vi "WILT.vi"() -> ()   [LabVIEW 2016] (continued)
"Temperature  Deg F (TC)"=0.0, "Volts"=0.0, "Volts (208)"=0.0, "SW (208)"=0.0}}, {"Lab ID"="", "Day Cycle Count"=0, "Station Label"="", "Dryer Details"={"Station"="", "Lab ID"="", "TR Number"=""}, "Status Color"=0, "Invisible Button"=FALSE, "Night Cycle Count"=0, "Station Index"=0, "Cycle Index"="", "Audit Alert"=FALSE, "Agilent Channel Definition"={"Channel"="", "Station"="", "Label"="", "Agilent Station"="", "Data"=0.0}, "DAQ Data"={"L1 Current"=0.0, "L2 Current"=0.0, "Temperature  Deg F (TC)"=0.0, "Volts"=0.0, "Volts (208)"=0.0, "SW (208)"=0.0}}, {"Lab ID"="", "Day Cycle Count"=0, "Station Label"="", "Dryer Details"={"Station"="", "Lab ID"="", "TR Number"=""}, "Status Color"=0, "Invisible Button"=FALSE, "Night Cycle Count"=0, "Station Index"=0, "Cycle Index"="", "Audit Alert"=FALSE, "Agilent Channel Definition"={"Channel"="", "Station"="", "Label"="", "Agilent Station"="", "Data"=0.0}, "DAQ Data"={"L1 Current"=0.0, "L2 Current"=0.0, "Temperature  Deg F (TC)"=0.0, "Volts"=0.0, "Volts (208)"=0.0, "SW (208)"=0.0}}] ("GUI Aisle 4_Const")) -> (w1:T3[])
  n20 = call <vilib>:"Add State(s) to Queue__jki_lib_state_machine.vi"("State(s) in (\"\")"=w59) -> ("States Out"=w60:string)  [unwired: 14 in]
  n21 = Create User Event(user event datatype=w46) -> (user event=w44:refnum<user-event>, error out=w41:errorcluster)  [unwired: 1 in]
  n22 = Obtain Notifier(name (unnamed)="GUI Aisle", notification data type=w1, error in (no error)=w34) -> (notifier out=w29:refnum<notifier>, error out=w33:errorcluster)  [unwired: 1 in, 1 out]
  n23 = while "Main Control SM" {
    shift-right: [w91] -> _
    shift-left: _ -> [w90]
    shift-right: [w93] -> w31
    shift-left: w33 -> [w88]
    shift-right: [w92] -> _
    shift-left: w60 -> [w94]
    shift-right: [w85] -> _
    shift-left: string[] [] -> [w86]
    tunnel: w29 -> [w82]
    tunnel: [w81] -> w32
    tunnel: w2 -> [w80]
    stop <- w87 stop-if-true
    # "Main Control SM"
    n24 = call <vilib>:"Parse State Queue__jki_lib_state_machine.vi"("State Queue"=w94, "Error In (no error)"=w88) -> ("Remaining States"=w96:string, "Current State"=w84:string, "Arguments"=w95:string)  [unwired: 11 in]
    n25 = case shown="\"Station 42\"" w84 {
      selector: w84 -> [_ _ w2449 _ _ _ _ _ _ _ _ _ _ _ _ _ _ _ _ _ _ _ _ _ _ _ _ _ _ _ _ _ _ _ _ _ _ _ _ _ _ _ _ _ _ _ _ _ _ _ _ _ _ _ _ _ _ _ _ _ _ _ _ _ _ _ _ _ _ _ _ _ _ _ _ _ _ _ _ _ _ _ _ _ _ _ _ _]
      tunnel: w96 -> [w116 w2447 w2453 w2472 w2479 w2485 w2490 w2514 w2521 w2526 w2544 w2563 w2582 w2590 w2597 w2609 w2644 w2661 w2688 w2700 w2709 w2718 w2725 w2730 w2736 w2747 w2752 w2761 w2788 w2815 w2842 w2869 w2896 w2923 w2950 w2977 w3004 w3031 w3058 w3085 w3112 w3139 w3166 w3193 w3220 w3247 w3274 w3301 w3328 w3355 w3382 w3409 w3436 w3463 w3490 w3517 w3544 w3571 w3598 w3625 w3652 w3679 w3706 w3733 w3760 w3787 w3814 w3841 w3868 w3895 w3922 w3949 w3976 w4003 w4030 w4057 w4084 w4111 w4138 w4165 w4192 w4219 w4246 w4273 w4295 w4319 w4348 w4352]
      tunnel: w95 -> [_ _ _ _ _ _ _ _ _ _ _ _ _ _ w2592 w2603 _ _ _ _ _ _ _ _ _ _ _ _ _ _ _ _ _ _ _ _ _ _ _ _ _ _ _ _ _ _ _ _ _ _ _ _ _ _ _ _ _ _ _ _ _ _ _ _ _ _ _ _ _ _ _ _ _ _ _ _ _ _ _ _ _ _ _ _ _ _ _ _]
      tunnel: w90 -> [w114 w2444 w2451 w2463 w2476 w2483 w2487 _ w2516 w2523 w2533 w2555 w2571 w2586 w2595 w2605 w2637 w2645 w2683 w2696 w2705 w2714 w2722 w2727 w2733 w2744 w2749 w2757 w2786 w2813 w2840 w2867 w2894 w2921 w2948 w2975 w3002 w3029 w3056 w3083 w3110 w3137 w3164 w3191 w3218 w3245 w3272 w3299 w3326 w3353 w3380 w3407 w3434 w3461 w3488 w3515 w3542 w3569 w3596 w3623 w3650 w3677 w3704 w3731 w3758 w3785 w3812 w3839 w3866 w3893 w3920 w3947 w3974 w4001 w4028 w4055 w4082 w4109 w4136 w4163 w4190 w4217 w4244 w4271 w4291 w4317 w4346 w4353]
      tunnel: [w113 w2445 w2455 w2469 errorcluster {"status"=FALSE, "code"=0, "source"=""} ("error out") w2482 w2488 w2491 w2517 w2524 w2529 w2558 w2577 w2588 w2593 w2606 w2640 w2659 w2684 w2689 w2706 w2715 w2720 w2728 w2734 w2745 w2750 w2759 w2780 w2807 w2834 w2861 w2888 w2915 w2942 w2969 w2996 w3023 w3050 w3077 w3105 w3131 w3158 w3185 w3212 w3239 w3266 w3293 w3320 w3347 w3374 w3401 w3428 w3455 w3482 w3509 w3536 w3563 w3590 w3617 w3644 w3671 w3698 w3725 w3752 w3779 w3806 w3833 w3860 w3887 w3914 w3941 w3968 w3995 w4022 w4049 w4076 w4103 w4130 w4157 w4184 w4211 w4238 w4265 w4292 w4314 w4339 w4355] -> w93
      tunnel: w88 -> [w112 w2445 w2454 w2469 w2475 w2482 w2488 w2491 w2518 w2524 w2530 w2559 w2578 w2588 w2594 w2607 w2641 w2659 w2685 w2690 w2706 w2715 w2721 w2728 w2734 w2745 w2750 w2759 w2781 w2808 w2835 w2862 w2889 w2916 w2943 w2970 w2997 w3024 w3051 w3078 w3106 w3132 w3159 w3186 w3213 w3240 w3267 w3294 w3321 w3348 w3375 w3402 w3429 w3456 w3483 w3510 w3537 w3564 w3591 w3618 w3645 w3672 w3699 w3726 w3753 w3780 w3807 w3834 w3861 w3888 w3915 w3942 w3969 w3996 w4023 w4050 w4077 w4104 w4131 w4158 w4185 w4212 w4239 w4266 w4279 w4316 w4339 w4355]
      tunnel: [w115 w2446 w2452 w2471 w2478 w2484 w2489 w2513 w2520 w2525 w2543 w2562 w2581 w2589 w2596 w2608 w2643 w2660 w2687 w2699 w2708 w2717 w2724 w2729 w2735 w2746 w2751 w2760 w2787 w2814 w2841 w2868 w2895 w2922 w2949 w2976 w3003 w3030 w3057 w3084 w3111 w3138 w3165 w3192 w3219 w3246 w3273 w3300 w3327 w3354 w3381 w3408 w3435 w3462 w3489 w3516 w3543 w3570 w3597 w3624 w3651 w3678 w3705 w3732 w3759 w3786 w3813 w3840 w3867 w3894 w3921 w3948 w3975 w4002 w4029 w4056 w4083 w4110 w4137 w4164 w4191 w4218 w4245 w4272 w4294 w4318 w4347 w4351] -> w92
      tunnel: [_ _ _ _ _ TRUE _ _ _ _ _ _ _ _ _ _ _ _ _ _ _ _ _ _ _ _ _ _ _ _ _ _ _ _ _ _ _ _ _ _ _ _ _ _ _ _ _ _ _ _ _ _ _ _ _ _ _ _ _ _ _ _ _ _ _ _ _ _ _ _ _ _ _ _ _ _ _ _ _ _ _ _ _ _ _ _ _ _] -> w87
      tunnel: [w111 w2444 w2451 w2470 w2476 w2483 w2487 w2492 w2516 w2523 w2542 w2561 w2580 w2586 w2595 w2605 w2636 w2652 w2683 w2696 w2704 w2713 w2722 w2727 w2733 w2744 w2749 w2756 w2785 w2812 w2839 w2866 w2893 w2920 w2947 w2974 w3001 w3028 w3055 w3082 w3109 w3136 w3163 w3190 w3217 w3244 w3271 w3298 w3325 w3352 w3379 w3406 w3433 w3460 w3487 w3514 w3541 w3568 w3595 w3622 w3649 w3676 w3703 w3730 w3757 w3784 w3811 w3838 w3865 w3892 w3919 w3946 w3973 w4000 w4027 w4054 w4081 w4108 w4135 w4162 w4189 w4216 w4243 w4270 w4293 w4317 w4346 w4354] -> w91
      tunnel: 500 ("Timeout") -> [w110 _ _ _ _ _ _ _ _ _ _ _ _ _ _ _ _ _ _ _ _ _ _ _ _ _ _ _ _ _ _ _ _ _ _ _ _ _ _ _ _ _ _ _ _ _ _ _ _ _ _ _ _ _ _ _ _ _ _ _ _ _ _ _ _ _ _ _ _ _ _ _ _ _ _ _ _ _ _ _ _ _ _ _ _ _ _ _]
      tunnel: w82 -> [w109 w2443 w2448 w2460 w2473 w2480 w2486 w2503 w2515 w2522 w2534 w2560 w2565 w2583 w2591 w2602 w2638 w2650 w2686 w2697 w2707 w2716 w2723 w2726 w2731 w2737 w2748 w2758 w2776 w2803 w2830 w2857 w2884 w2911 w2938 w2965 w2992 w3019 w3046 w3073 w3101 w3127 w3154 w3181 w3208 w3235 w3262 w3289 w3316 w3343 w3370 w3397 w3424 w3451 w3478 w3505 w3532 w3559 w3586 w3613 w3640 w3667 w3694 w3721 w3748 w3775 w3802 w3829 w3856 w3883 w3910 w3937 w3964 w3991 w4018 w4045 w4072 w4099 w4126 w4153 w4180 w4207 w4234 w4261 w4280 w4304 w4345 w4349]
      tunnel: [w109 w2443 w2448 w2460 w2473 w2480 w2486 w2503 w2515 w2522 w2534 w2560 w2565 w2583 w2591 w2602 w2638 w2650 w2686 w2697 w2707 w2716 w2723 w2726 w2731 w2737 w2748 w2758 w2776 w2803 w2830 w2857 w2884 w2911 w2938 w2965 w2992 w3019 w3046 w3073 w3101 w3127 w3154 w3181 w3208 w3235 w3262 w3289 w3316 w3343 w3370 w3397 w3424 w3451 w3478 w3505 w3532 w3559 w3586 w3613 w3640 w3667 w3694 w3721 w3748 w3775 w3802 w3829 w3856 w3883 w3910 w3937 w3964 w3991 w4018 w4045 w4072 w4099 w4126 w4153 w4180 w4207 w4234 w4261 w4280 w4302 w4345 w4349] -> w81
      tunnel: w80 -> [w108 _ _ _ _ _ _ _ _ _ _ _ _ _ _ _ _ _ _ _ _ _ _ _ _ _ _ _ _ _ _ _ _ _ _ _ _ _ _ _ _ _ _ _ _ _ _ _ _ _ _ _ _ _ _ _ _ _ _ _ _ _ _ _ _ _ _ _ _ _ _ _ _ _ _ _ _ _ _ _ _ _ _ _ _ _ _ _]
      frame "", "Idle" {
        n26 = event shown="[113] <Aisle 1 Update>: User Event" {
          selector: w108 -> [_ _ _ _ _ _ _ _ _ _ _ _ _ _ _ _ _ _ _ _ _ _ _ _ _ _ _ _ _ _ _ _ _ _ _ _ _ _ _ _ _ _ _ _ _ _ _ _ _ _ _ _ _ _ _ _ _ _ _ _ _ _ _ _ _ _ _ _ _ _ _ _ _ _ _ _ _ _ _ _ _ _ _ _ _ _ _ _ _ _ _ _ _ _ _ _ _ _ _ _ _ _ _ _ _ _ _ _ _ _ _ _ _ _ _ _ _ _ _ _ _ _ _ _]
          dyn-events: _ -> [_ _ _ _ _ _ _ _ _ _ _ _ _ _ _ _ _ _ _ _ _ _ _ _ _ _ _ _ _ _ _ _ _ _ _ _ _ _ _ _ _ _ _ _ _ _ _ _ _ _ _ _ _ _ _ _ _ _ _ _ _ _ _ _ _ _ _ _ _ _ _ _ _ _ _ _ _ _ _ _ _ _ _ _ _ _ _ _ _ _ _ _ _ _ _ _ _ _ _ _ _ _ _ _ _ _ _ _ _ _ _ _ _ _ _ _ _ _ _ _ _ _ _ _]
          timeout: w110 -> [_ _ _ _ _ _ _ _ _ _ _ _ _ _ _ _ _ _ _ _ _ _ _ _ _ _ _ _ _ _ _ _ _ _ _ _ _ _ _ _ _ _ _ _ _ _ _ _ _ _ _ _ _ _ _ _ _ _ _ _ _ _ _ _ _ _ _ _ _ _ _ _ _ _ _ _ _ _ _ _ _ _ _ _ _ _ _ _ _ _ _ _ _ _ _ _ _ _ _ _ _ _ _ _ _ _ _ _ _ _ _ _ _ _ _ _ _ _ _ _ _ _ _ _]
          tunnel: w116 -> [w121 w127 w147 w167 w187 w207 w227 w247 w267 w287 w307 w327 w347 w367 w387 w407 w427 w447 w467 w487 w507 w527 w547 w567 w587 w607 w627 w647 w667 w687 w707 w727 w747 w767 w787 w807 w827 w847 w867 w887 w907 w927 w947 w967 w987 w1007 w1027 w1047 w1067 w1087 w1107 w1127 w1147 w1167 w1187 w1207 w1227 w1247 w1267 w1287 w1307 w1327 w1347 w1367 w1387 w1407 w1427 w1447 w1467 w1487 w1507 w1527 w1556 w1562 w1582 w1602 w1622 w1642 w1662 w1682 w1702 w1722 w1742 w1762 w1782 w1802 w1822 w1842 w1862 w1882 w1902 w1922 w1942 w1962 w1982 w2002 w2022 w2042 w2062 w2082 w2102 w2122 w2142 w2162 w2182 w2202 w2222 w2242 w2262 w2282 w2302 w2322 w2342 w2363 w2372 w2380 w2388 w2395 w2400 w2408 w2417 w2426 w2436 w2442]
          tunnel: [w119 w126 w146 w166 w186 w206 w226 w246 w266 w286 w306 w326 w346 w366 w386 w406 w426 w446 w466 w486 w506 w526 w546 w566 w586 w606 w626 w646 w666 w686 w706 w726 w746 w766 w786 w806 w826 w846 w866 w886 w906 w926 w946 w966 w986 w1006 w1026 w1046 w1066 w1086 w1106 w1126 w1146 w1166 w1186 w1206 w1226 w1246 w1266 w1286 w1306 w1326 w1346 w1366 w1386 w1406 w1426 w1446 w1466 w1486 w1506 w1526 w1555 w1561 w1581 w1601 w1621 w1641 w1661 w1681 w1701 w1721 w1741 w1761 w1781 w1801 w1821 w1841 w1861 w1881 w1901 w1921 w1941 w1961 w1981 w2001 w2021 w2041 w2061 w2081 w2101 w2121 w2141 w2161 w2181 w2201 w2221 w2241 w2261 w2281 w2301 w2321 w2341 w2363 w2372 w2380 w2388 w2395 w2399 w2407 w2418 w2427 w2435 w2441] -> w115
          tunnel: w114 -> [w118 w125 w145 w165 w185 w205 w225 w245 w265 w285 w305 w325 w345 w365 w385 w405 w425 w445 w465 w485 w505 w525 w545 w565 w585 w605 w625 w645 w665 w685 w705 w725 w745 w765 w785 w805 w825 w845 w865 w885 w905 w925 w945 w965 w985 w1005 w1025 w1045 w1065 w1085 w1105 w1125 w1145 w1165 w1185 w1205 w1225 w1245 w1265 w1285 w1305 w1325 w1345 w1365 w1385 w1405 w1425 w1445 w1465 w1485 w1505 w1525 w1551 w1560 w1580 w1600 w1620 w1640 w1660 w1680 w1700 w1720 w1740 w1760 w1780 w1800 w1820 w1840 w1860 w1880 w1900 w1920 w1940 w1960 w1980 w2000 w2020 w2040 w2060 w2080 w2100 w2120 w2140 w2160 w2180 w2200 w2220 w2240 w2260 w2280 w2300 w2320 w2340 w2362 w2370 w2378 w2386 w2394 w2401 w2409 w2419 w2428 w2433 w2439]
          tunnel: [w120 w123 w143 w163 w183 w203 w223 w243 w263 w283 w303 w323 w343 w363 w383 w403 w423 w443 w463 w483 w503 w523 w543 w563 w583 w603 w624 w643 w663 w683 w703 w723 w743 w763 w783 w803 w823 w843 w863 w883 w903 w923 w943 w963 w983 w1003 w1023 w1043 w1063 w1083 w1103 w1123 w1143 w1163 w1183 w1203 w1223 w1243 w1263 w1283 w1303 w1323 w1343 w1363 w1383 w1403 w1423 w1443 w1463 w1483 w1503 w1523 w1548 w1558 w1578 w1598 w1618 w1638 w1658 w1678 w1698 w1718 w1738 w1758 w1778 w1798 w1818 w1838 w1858 w1878 w1898 w1918 w1938 w1958 w1978 w1998 w2018 w2038 w2058 w2078 w2098 w2118 w2138 w2158 w2178 w2198 w2218 w2238 w2258 w2278 w2298 w2318 w2338 w2364 w2371 w2379 w2387 w2396 w2402 w2410 w2416 w2425 w2434 w2440] -> w113
          tunnel: w112 -> [w120 w124 w144 w164 w184 w204 w224 w244 w264 w284 w304 w324 w344 w364 w384 w404 w424 w444 w464 w484 w504 w524 w544 w564 w584 w604 w623 w644 w664 w684 w704 w724 w744 w764 w784 w804 w824 w844 w864 w884 w904 w924 w944 w964 w984 w1004 w1024 w1044 w1064 w1084 w1104 w1124 w1144 w1164 w1184 w1204 w1224 w1244 w1264 w1284 w1304 w1324 w1344 w1364 w1384 w1404 w1424 w1444 w1464 w1484 w1504 w1524 w1549 w1559 w1579 w1599 w1619 w1639 w1659 w1679 w1699 w1719 w1739 w1759 w1779 w1799 w1819 w1839 w1859 w1879 w1899 w1919 w1939 w1959 w1979 w1999 w2019 w2039 w2059 w2079 w2099 w2119 w2139 w2159 w2179 w2199 w2219 w2239 w2259 w2279 w2299 w2319 w2339 w2364 w2371 w2379 w2387 w2396 w2402 w2410 w2416 w2425 w2434 w2440]
          tunnel: [w118 w125 w145 w165 w185 w205 w225 w245 w265 w285 w305 w325 w345 w365 w385 w405 w425 w445 w465 w485 w505 w525 w545 w565 w585 w605 w625 w645 w665 w685 w705 w725 w745 w765 w785 w805 w825 w845 w865 w885 w905 w925 w945 w965 w985 w1005 w1025 w1045 w1065 w1085 w1105 w1125 w1145 w1165 w1185 w1205 w1225 w1245 w1265 w1285 w1305 w1325 w1345 w1365 w1385 w1405 w1425 w1445 w1465 w1485 w1505 w1525 w1551 w1560 w1580 w1600 w1620 w1640 w1660 w1680 w1700 w1720 w1740 w1760 w1780 w1800 w1820 w1840 w1860 w1880 w1900 w1920 w1940 w1960 w1980 w2000 w2020 w2040 w2060 w2080 w2100 w2120 w2140 w2160 w2180 w2200 w2220 w2240 w2260 w2280 w2300 w2320 w2340 w2361 w2369 w2377 w2385 w2393 w2401 w2409 w2419 w2428 w2433 w2439] -> w111
          event Timeout {
            n27 = event-data() -> ()  [unwired: 1 in, 1 out]
            n28 = Unbundle By Name(w118) -> ("States"=w117:string)
            n29 = call <vilib>:"Add State(s) to Queue__jki_lib_state_machine.vi"("State(s) in Front (\"\")"=w117, "State(s) in (\"\")"=w121) -> ("States Out"=w119:string)  [unwired: 13 in]
          }
          event Value Change {
            n30 = event-data() -> ("NewVal"=w122:bool)  [unwired: 1 in, 2 out]
            n31 = case shown="True" w122 {
              tunnel: w125 -> [_ w138]
              tunnel: w124 -> [w128 w136]
              tunnel: [w128 w135] -> w123
              tunnel: w122 -> [_ w134]
              frame False {
              }
              frame True {
                n32 = local read "Agilent Semaphore"() -> (w139:T1[])
                n33 = Unbundle By Name(w138) -> ("Agilent Switches"=w137:T2[])
                n34 = Number To Decimal String(number=1) -> (decimal integer string=w141:string)  [unwired: 1 in]
                n35 = Not(x=w134) -> (.not. x?=w140:bool)
                n36 = call "WILT Agilent Valve Control.vi"("Station In"=w141, "Agilent Channels In"=w137, "Semaphore"=w139, "Search"=T19 "Water Valve", "Open/Close (F:Close)"=w140, "error in (no error)"=w136, "Test Type"="Test Type", "Number Of Cycles"="Number of ON/OFF Cycles", "Cycle Time (mS)"="Valve ON Time (mS)") -> ("error out"=w135:errorcluster)  [unwired: 4 in, 2 out]
              }
            }
            n37 = call <vilib>:"Add State(s) to Queue__jki_lib_state_machine.vi"("State(s) in (\"\")"=w127) -> ("States Out"=w126:string)  [unwired: 14 in]
          }
          event Value Change {
            n38 = event-data() -> ("NewVal"=w142:bool)  [unwired: 1 in, 2 out]
            n39 = case shown="False" w142 {
              tunnel: w145 -> [_ w158]
              tunnel: w144 -> [w148 w156]
              tunnel: [w148 w155] -> w143
              tunnel: w142 -> [_ w154]
              frame False {
              }
              frame True {
                n40 = local read "Number of ON/OFF Cycles"() -> (w150:i32)
                n41 = local read "Valve ON Time (mS)"() -> (w149:u32)
                n42 = local read "Agilent Semaphore"() -> (w159:T1[])
                n43 = Unbundle By Name(w158) -> ("Agilent Switches"=w157:T2[])
                n44 = local read "Test Type"() -> (w151:T12)
                n45 = Number To Decimal String(number=2) -> (decimal integer string=w161:string)  [unwired: 1 in]
                n46 = Not(x=w154) -> (.not. x?=w160:bool)
                n47 = call "WILT Agilent Valve Control.vi"("Station In"=w161, "Agilent Channels In"=w157, "Semaphore"=w159, "Search"=T19 "Water Valve", "Open/Close (F:Close)"=w160, "error in (no error)"=w156, "Test Type"=w151, "Number Of Cycles"=w150, "Cycle Time (mS)"=w149) -> ("error out"=w155:errorcluster)  [unwired: 4 in, 2 out]
              }
            }
            n48 = call <vilib>:"Add State(s) to Queue__jki_lib_state_machine.vi"("State(s) in (\"\")"=w147) -> ("States Out"=w146:string)  [unwired: 14 in]
          }
          event Value Change {
            n49 = event-data() -> ("NewVal"=w162:bool)  [unwired: 1 in, 2 out]
            n50 = case shown="True" w162 {
              tunnel: w165 -> [_ w178]
              tunnel: w164 -> [w168 w176]
              tunnel: [w168 w175] -> w163
              tunnel: w162 -> [_ w174]
              frame False {
              }
              frame True {
                n51 = local read "Number of ON/OFF Cycles"() -> (w170:i32)
                n52 = local read "Valve ON Time (mS)"() -> (w169:u32)
                n53 = local read "Agilent Semaphore"() -> (w179:T1[])
                n54 = Unbundle By Name(w178) -> ("Agilent Switches"=w177:T2[])
                n55 = local read "Test Type"() -> (w171:T12)
                n56 = Number To Decimal String(number=3) -> (decimal integer string=w181:string)  [unwired: 1 in]
                n57 = Not(x=w174) -> (.not. x?=w180:bool)
                n58 = call "WILT Agilent Valve Control.vi"("Station In"=w181, "Agilent Channels In"=w177, "Semaphore"=w179, "Search"=T19 "Water Valve", "Open/Close (F:Close)"=w180, "error in (no error)"=w176, "Test Type"=w171, "Number Of Cycles"=w170, "Cycle Time (mS)"=w169) -> ("error out"=w175:errorcluster)  [unwired: 4 in, 2 out]
              }
            }
            n59 = call <vilib>:"Add State(s) to Queue__jki_lib_state_machine.vi"("State(s) in (\"\")"=w167) -> ("States Out"=w166:string)  [unwired: 14 in]
          }
          event Value Change {
            n60 = event-data() -> ("NewVal"=w182:bool)  [unwired: 1 in, 2 out]
            n61 = case shown="True" w182 {
              tunnel: w185 -> [_ w198]
              tunnel: w184 -> [w188 w196]
              tunnel: [w188 w195] -> w183
              tunnel: w182 -> [_ w194]
              frame False {
              }
              frame True {
                n62 = local read "Number of ON/OFF Cycles"() -> (w190:i32)
                n63 = local read "Valve ON Time (mS)"() -> (w189:u32)
                n64 = local read "Agilent Semaphore"() -> (w199:T1[])
                n65 = Unbundle By Name(w198) -> ("Agilent Switches"=w197:T2[])
                n66 = local read "Test Type"() -> (w191:T12)
                n67 = Number To Decimal String(number=4) -> (decimal integer string=w201:string)  [unwired: 1 in]
                n68 = Not(x=w194) -> (.not. x?=w200:bool)
                n69 = call "WILT Agilent Valve Control.vi"("Station In"=w201, "Agilent Channels In"=w197, "Semaphore"=w199, "Search"=T19 "Water Valve", "Open/Close (F:Close)"=w200, "error in (no error)"=w196, "Test Type"=w191, "Number Of Cycles"=w190, "Cycle Time (mS)"=w189) -> ("error out"=w195:errorcluster)  [unwired: 4 in, 2 out]
              }
            }
            n70 = call <vilib>:"Add State(s) to Queue__jki_lib_state_machine.vi"("State(s) in (\"\")"=w187) -> ("States Out"=w186:string)  [unwired: 14 in]
          }
          event Value Change {
            n71 = event-data() -> ("NewVal"=w202:bool)  [unwired: 1 in, 2 out]
            n72 = case shown="True" w202 {
              tunnel: w205 -> [_ w218]
              tunnel: w204 -> [w208 w216]
              tunnel: [w208 w215] -> w203
              tunnel: w202 -> [_ w214]
              frame False {
              }
              frame True {
                n73 = local read "Number of ON/OFF Cycles"() -> (w210:i32)
                n74 = local read "Valve ON Time (mS)"() -> (w209:u32)
                n75 = local read "Agilent Semaphore"() -> (w219:T1[])
                n76 = Unbundle By Name(w218) -> ("Agilent Switches"=w217:T2[])
                n77 = local read "Test Type"() -> (w211:T12)
                n78 = Number To Decimal String(number=5) -> (decimal integer string=w221:string)  [unwired: 1 in]
                n79 = Not(x=w214) -> (.not. x?=w220:bool)
                n80 = call "WILT Agilent Valve Control.vi"("Station In"=w221, "Agilent Channels In"=w217, "Semaphore"=w219, "Search"=T19 "Water Valve", "Open/Close (F:Close)"=w220, "error in (no error)"=w216, "Test Type"=w211, "Number Of Cycles"=w210, "Cycle Time (mS)"=w209) -> ("error out"=w215:errorcluster)  [unwired: 4 in, 2 out]
              }
            }
            n81 = call <vilib>:"Add State(s) to Queue__jki_lib_state_machine.vi"("State(s) in (\"\")"=w207) -> ("States Out"=w206:string)  [unwired: 14 in]
          }
          event Value Change {
            n82 = event-data() -> ("NewVal"=w222:bool)  [unwired: 1 in, 2 out]
            n83 = case shown="True" w222 {
              tunnel: w225 -> [_ w238]
              tunnel: w224 -> [w228 w236]
              tunnel: [w228 w235] -> w223
              tunnel: w222 -> [_ w234]
              frame False {
              }
              frame True {
                n84 = local read "Number of ON/OFF Cycles"() -> (w230:i32)
                n85 = local read "Valve ON Time (mS)"() -> (w229:u32)
                n86 = local read "Agilent Semaphore"() -> (w239:T1[])
                n87 = Unbundle By Name(w238) -> ("Agilent Switches"=w237:T2[])
                n88 = local read "Test Type"() -> (w231:T12)
                n89 = Number To Decimal String(number=6) -> (decimal integer string=w241:string)  [unwired: 1 in]
                n90 = Not(x=w234) -> (.not. x?=w240:bool)
                n91 = call "WILT Agilent Valve Control.vi"("Station In"=w241, "Agilent Channels In"=w237, "Semaphore"=w239, "Search"=T19 "Water Valve", "Open/Close (F:Close)"=w240, "error in (no error)"=w236, "Test Type"=w231, "Number Of Cycles"=w230, "Cycle Time (mS)"=w229) -> ("error out"=w235:errorcluster)  [unwired: 4 in, 2 out]
              }
            }
            n92 = call <vilib>:"Add State(s) to Queue__jki_lib_state_machine.vi"("State(s) in (\"\")"=w227) -> ("States Out"=w226:string)  [unwired: 14 in]
          }
          event Value Change {
            n93 = event-data() -> ("NewVal"=w242:bool)  [unwired: 1 in, 2 out]
            n94 = case shown="True" w242 {
              tunnel: w245 -> [_ w258]
              tunnel: w244 -> [w248 w256]
              tunnel: [w248 w255] -> w243
              tunnel: w242 -> [_ w254]
              frame False {
              }
              frame True {
                n95 = local read "Number of ON/OFF Cycles"() -> (w250:i32)
                n96 = local read "Valve ON Time (mS)"() -> (w249:u32)
                n97 = local read "Agilent Semaphore"() -> (w259:T1[])
                n98 = Unbundle By Name(w258) -> ("Agilent Switches"=w257:T2[])
                n99 = local read "Test Type"() -> (w251:T12)
                n100 = Number To Decimal String(number=7) -> (decimal integer string=w261:string)  [unwired: 1 in]
                n101 = Not(x=w254) -> (.not. x?=w260:bool)
                n102 = call "WILT Agilent Valve Control.vi"("Station In"=w261, "Agilent Channels In"=w257, "Semaphore"=w259, "Search"=T19 "Water Valve", "Open/Close (F:Close)"=w260, "error in (no error)"=w256, "Test Type"=w251, "Number Of Cycles"=w250, "Cycle Time (mS)"=w249) -> ("error out"=w255:errorcluster)  [unwired: 4 in, 2 out]
              }
            }
            n103 = call <vilib>:"Add State(s) to Queue__jki_lib_state_machine.vi"("State(s) in (\"\")"=w247) -> ("States Out"=w246:string)  [unwired: 14 in]
          }
          event Value Change {
            n104 = event-data() -> ("NewVal"=w262:bool)  [unwired: 1 in, 2 out]
            n105 = case shown="True" w262 {
              tunnel: w265 -> [_ w278]
              tunnel: w264 -> [w268 w276]
              tunnel: [w268 w275] -> w263
              tunnel: w262 -> [_ w274]
              frame False {
              }
              frame True {
                n106 = local read "Number of ON/OFF Cycles"() -> (w270:i32)
                n107 = local read "Valve ON Time (mS)"() -> (w269:u32)
                n108 = local read "Agilent Semaphore"() -> (w279:T1[])
                n109 = Unbundle By Name(w278) -> ("Agilent Switches"=w277:T2[])
                n110 = local read "Test Type"() -> (w271:T12)
                n111 = Number To Decimal String(number=8) -> (decimal integer string=w281:string)  [unwired: 1 in]
                n112 = Not(x=w274) -> (.not. x?=w280:bool)
                n113 = call "WILT Agilent Valve Control.vi"("Station In"=w281, "Agilent Channels In"=w277, "Semaphore"=w279, "Search"=T19 "Water Valve", "Open/Close (F:Close)"=w280, "error in (no error)"=w276, "Test Type"=w271, "Number Of Cycles"=w270, "Cycle Time (mS)"=w269) -> ("error out"=w275:errorcluster)  [unwired: 4 in, 2 out]
              }
            }
            n114 = call <vilib>:"Add State(s) to Queue__jki_lib_state_machine.vi"("State(s) in (\"\")"=w267) -> ("States Out"=w266:string)  [unwired: 14 in]
          }
          event Value Change {
            n115 = event-data() -> ("NewVal"=w282:bool)  [unwired: 1 in, 2 out]
            n116 = case shown="True" w282 {
              tunnel: w285 -> [_ w298]
              tunnel: w284 -> [w288 w296]
              tunnel: [w288 w295] -> w283
              tunnel: w282 -> [_ w294]
              frame False {
              }
              frame True {
                n117 = local read "Number of ON/OFF Cycles"() -> (w290:i32)
                n118 = local read "Valve ON Time (mS)"() -> (w289:u32)
                n119 = local read "Agilent Semaphore"() -> (w299:T1[])
                n120 = Unbundle By Name(w298) -> ("Agilent Switches"=w297:T2[])
                n121 = local read "Test Type"() -> (w291:T12)
                n122 = Number To Decimal String(number=9) -> (decimal integer string=w301:string)  [unwired: 1 in]
                n123 = Not(x=w294) -> (.not. x?=w300:bool)
                n124 = call "WILT Agilent Valve Control.vi"("Station In"=w301, "Agilent Channels In"=w297, "Semaphore"=w299, "Search"=T19 "Water Valve", "Open/Close (F:Close)"=w300, "error in (no error)"=w296, "Test Type"=w291, "Number Of Cycles"=w290, "Cycle Time (mS)"=w289) -> ("error out"=w295:errorcluster)  [unwired: 4 in, 2 out]
              }
            }
            n125 = call <vilib>:"Add State(s) to Queue__jki_lib_state_machine.vi"("State(s) in (\"\")"=w287) -> ("States Out"=w286:string)  [unwired: 14 in]
          }
          event Value Change {
            n126 = event-data() -> ("NewVal"=w302:bool)  [unwired: 1 in, 2 out]
            n127 = case shown="False" w302 {
              tunnel: w305 -> [_ w318]
              tunnel: w304 -> [w308 w316]
              tunnel: [w308 w315] -> w303
              tunnel: w302 -> [_ w314]
              frame False {
              }
              frame True {
                n128 = local read "Number of ON/OFF Cycles"() -> (w310:i32)
                n129 = local read "Valve ON Time (mS)"() -> (w309:u32)
                n130 = local read "Agilent Semaphore"() -> (w319:T1[])
                n131 = Unbundle By Name(w318) -> ("Agilent Switches"=w317:T2[])
                n132 = local read "Test Type"() -> (w311:T12)
                n133 = Number To Decimal String(number=10) -> (decimal integer string=w321:string)  [unwired: 1 in]
                n134 = Not(x=w314) -> (.not. x?=w320:bool)
                n135 = call "WILT Agilent Valve Control.vi"("Station In"=w321, "Agilent Channels In"=w317, "Semaphore"=w319, "Search"=T19 "Water Valve", "Open/Close (F:Close)"=w320, "error in (no error)"=w316, "Test Type"=w311, "Number Of Cycles"=w310, "Cycle Time (mS)"=w309) -> ("error out"=w315:errorcluster)  [unwired: 4 in, 2 out]
              }
            }
            n136 = call <vilib>:"Add State(s) to Queue__jki_lib_state_machine.vi"("State(s) in (\"\")"=w307) -> ("States Out"=w306:string)  [unwired: 14 in]
          }
          event Value Change {
            n137 = event-data() -> ("NewVal"=w322:bool)  [unwired: 1 in, 2 out]
            n138 = case shown="True" w322 {
              tunnel: w325 -> [_ w338]
              tunnel: w324 -> [w328 w336]
              tunnel: [w328 w335] -> w323
              tunnel: w322 -> [_ w334]
              frame False {
              }
              frame True {
                n139 = local read "Number of ON/OFF Cycles"() -> (w330:i32)
                n140 = local read "Valve ON Time (mS)"() -> (w329:u32)
                n141 = local read "Agilent Semaphore"() -> (w339:T1[])
                n142 = Unbundle By Name(w338) -> ("Agilent Switches"=w337:T2[])
                n143 = local read "Test Type"() -> (w331:T12)
                n144 = Number To Decimal String(number=11) -> (decimal integer string=w341:string)  [unwired: 1 in]
                n145 = Not(x=w334) -> (.not. x?=w340:bool)
                n146 = call "WILT Agilent Valve Control.vi"("Station In"=w341, "Agilent Channels In"=w337, "Semaphore"=w339, "Search"=T19 "Water Valve", "Open/Close (F:Close)"=w340, "error in (no error)"=w336, "Test Type"=w331, "Number Of Cycles"=w330, "Cycle Time (mS)"=w329) -> ("error out"=w335:errorcluster)  [unwired: 4 in, 2 out]
              }
            }
            n147 = call <vilib>:"Add State(s) to Queue__jki_lib_state_machine.vi"("State(s) in (\"\")"=w327) -> ("States Out"=w326:string)  [unwired: 14 in]
          }
          event Value Change {
            n148 = event-data() -> ("NewVal"=w342:bool)  [unwired: 1 in, 2 out]
            n149 = case shown="True" w342 {
              tunnel: w345 -> [_ w358]
              tunnel: w344 -> [w348 w356]
              tunnel: [w348 w355] -> w343
              tunnel: w342 -> [_ w354]
              frame False {
              }
              frame True {
                n150 = local read "Number of ON/OFF Cycles"() -> (w350:i32)
                n151 = local read "Valve ON Time (mS)"() -> (w349:u32)
                n152 = local read "Agilent Semaphore"() -> (w359:T1[])
                n153 = Unbundle By Name(w358) -> ("Agilent Switches"=w357:T2[])
                n154 = local read "Test Type"() -> (w351:T12)
                n155 = Number To Decimal String(number=12) -> (decimal integer string=w361:string)  [unwired: 1 in]
                n156 = Not(x=w354) -> (.not. x?=w360:bool)
                n157 = call "WILT Agilent Valve Control.vi"("Station In"=w361, "Agilent Channels In"=w357, "Semaphore"=w359, "Search"=T19 "Water Valve", "Open/Close (F:Close)"=w360, "error in (no error)"=w356, "Test Type"=w351, "Number Of Cycles"=w350, "Cycle Time (mS)"=w349) -> ("error out"=w355:errorcluster)  [unwired: 4 in, 2 out]
              }
            }
            n158 = call <vilib>:"Add State(s) to Queue__jki_lib_state_machine.vi"("State(s) in (\"\")"=w347) -> ("States Out"=w346:string)  [unwired: 14 in]
          }
          event Value Change {
            n159 = event-data() -> ("NewVal"=w362:bool)  [unwired: 1 in, 2 out]
            n160 = case shown="True" w362 {
              tunnel: w365 -> [_ w378]
              tunnel: w364 -> [w368 w376]
              tunnel: [w368 w375] -> w363
              tunnel: w362 -> [_ w374]
              frame False {
              }
              frame True {
                n161 = local read "Number of ON/OFF Cycles"() -> (w370:i32)
                n162 = local read "Valve ON Time (mS)"() -> (w369:u32)
                n163 = local read "Agilent Semaphore"() -> (w379:T1[])
                n164 = Unbundle By Name(w378) -> ("Agilent Switches"=w377:T2[])
                n165 = local read "Test Type"() -> (w371:T12)
                n166 = Number To Decimal String(number=13) -> (decimal integer string=w381:string)  [unwired: 1 in]
                n167 = Not(x=w374) -> (.not. x?=w380:bool)
                n168 = call "WILT Agilent Valve Control.vi"("Station In"=w381, "Agilent Channels In"=w377, "Semaphore"=w379, "Search"=T19 "Water Valve", "Open/Close (F:Close)"=w380, "error in (no error)"=w376, "Test Type"=w371, "Number Of Cycles"=w370, "Cycle Time (mS)"=w369) -> ("error out"=w375:errorcluster)  [unwired: 4 in, 2 out]
              }
            }
            n169 = call <vilib>:"Add State(s) to Queue__jki_lib_state_machine.vi"("State(s) in (\"\")"=w367) -> ("States Out"=w366:string)  [unwired: 14 in]
          }
          event Value Change {
            n170 = event-data() -> ("NewVal"=w382:bool)  [unwired: 1 in, 2 out]
            n171 = case shown="True" w382 {
              tunnel: w385 -> [_ w398]
              tunnel: w384 -> [w388 w396]
              tunnel: [w388 w395] -> w383
              tunnel: w382 -> [_ w394]
              frame False {
              }
              frame True {
                n172 = local read "Number of ON/OFF Cycles"() -> (w390:i32)
                n173 = local read "Valve ON Time (mS)"() -> (w389:u32)
                n174 = local read "Agilent Semaphore"() -> (w399:T1[])
                n175 = Unbundle By Name(w398) -> ("Agilent Switches"=w397:T2[])
                n176 = local read "Test Type"() -> (w391:T12)
                n177 = Number To Decimal String(number=14) -> (decimal integer string=w401:string)  [unwired: 1 in]
                n178 = Not(x=w394) -> (.not. x?=w400:bool)
                n179 = call "WILT Agilent Valve Control.vi"("Station In"=w401, "Agilent Channels In"=w397, "Semaphore"=w399, "Search"=T19 "Water Valve", "Open/Close (F:Close)"=w400, "error in (no error)"=w396, "Test Type"=w391, "Number Of Cycles"=w390, "Cycle Time (mS)"=w389) -> ("error out"=w395:errorcluster)  [unwired: 4 in, 2 out]
              }
            }
            n180 = call <vilib>:"Add State(s) to Queue__jki_lib_state_machine.vi"("State(s) in (\"\")"=w387) -> ("States Out"=w386:string)  [unwired: 14 in]
          }
          event Value Change {
            n181 = event-data() -> ("NewVal"=w402:bool)  [unwired: 1 in, 2 out]
            n182 = case shown="True" w402 {
              tunnel: w405 -> [_ w418]
              tunnel: w404 -> [w408 w416]
              tunnel: [w408 w415] -> w403
              tunnel: w402 -> [_ w414]
              frame False {
              }
              frame True {
                n183 = local read "Number of ON/OFF Cycles"() -> (w410:i32)
                n184 = local read "Valve ON Time (mS)"() -> (w409:u32)
                n185 = local read "Agilent Semaphore"() -> (w419:T1[])
                n186 = Unbundle By Name(w418) -> ("Agilent Switches"=w417:T2[])
                n187 = local read "Test Type"() -> (w411:T12)
                n188 = Number To Decimal String(number=15) -> (decimal integer string=w421:string)  [unwired: 1 in]
                n189 = Not(x=w414) -> (.not. x?=w420:bool)
                n190 = call "WILT Agilent Valve Control.vi"("Station In"=w421, "Agilent Channels In"=w417, "Semaphore"=w419, "Search"=T19 "Water Valve", "Open/Close (F:Close)"=w420, "error in (no error)"=w416, "Test Type"=w411, "Number Of Cycles"=w410, "Cycle Time (mS)"=w409) -> ("error out"=w415:errorcluster)  [unwired: 4 in, 2 out]
              }
            }
            n191 = call <vilib>:"Add State(s) to Queue__jki_lib_state_machine.vi"("State(s) in (\"\")"=w407) -> ("States Out"=w406:string)  [unwired: 14 in]
          }
          event Value Change {
            n192 = event-data() -> ("NewVal"=w422:bool)  [unwired: 1 in, 2 out]
            n193 = case shown="True" w422 {
              tunnel: w425 -> [_ w438]
              tunnel: w424 -> [w428 w436]
              tunnel: [w428 w435] -> w423
              tunnel: w422 -> [_ w434]
              frame False {
              }
              frame True {
                n194 = local read "Number of ON/OFF Cycles"() -> (w430:i32)
                n195 = local read "Valve ON Time (mS)"() -> (w429:u32)
                n196 = local read "Agilent Semaphore"() -> (w439:T1[])
                n197 = Unbundle By Name(w438) -> ("Agilent Switches"=w437:T2[])
                n198 = local read "Test Type"() -> (w431:T12)
                n199 = Number To Decimal String(number=16) -> (decimal integer string=w441:string)  [unwired: 1 in]
                n200 = Not(x=w434) -> (.not. x?=w440:bool)
                n201 = call "WILT Agilent Valve Control.vi"("Station In"=w441, "Agilent Channels In"=w437, "Semaphore"=w439, "Search"=T19 "Water Valve", "Open/Close (F:Close)"=w440, "error in (no error)"=w436, "Test Type"=w431, "Number Of Cycles"=w430, "Cycle Time (mS)"=w429) -> ("error out"=w435:errorcluster)  [unwired: 4 in, 2 out]
              }
            }
            n202 = call <vilib>:"Add State(s) to Queue__jki_lib_state_machine.vi"("State(s) in (\"\")"=w427) -> ("States Out"=w426:string)  [unwired: 14 in]
          }
          event Value Change {
            n203 = event-data() -> ("NewVal"=w442:bool)  [unwired: 1 in, 2 out]
            n204 = case shown="True" w442 {
              tunnel: w445 -> [_ w458]
              tunnel: w444 -> [w448 w456]
              tunnel: [w448 w455] -> w443
              tunnel: w442 -> [_ w454]
              frame False {
              }
              frame True {
                n205 = local read "Number of ON/OFF Cycles"() -> (w450:i32)
                n206 = local read "Valve ON Time (mS)"() -> (w449:u32)
                n207 = local read "Agilent Semaphore"() -> (w459:T1[])
                n208 = Unbundle By Name(w458) -> ("Agilent Switches"=w457:T2[])
                n209 = local read "Test Type"() -> (w451:T12)
                n210 = Number To Decimal String(number=17) -> (decimal integer string=w461:string)  [unwired: 1 in]
                n211 = Not(x=w454) -> (.not. x?=w460:bool)
                n212 = call "WILT Agilent Valve Control.vi"("Station In"=w461, "Agilent Channels In"=w457, "Semaphore"=w459, "Search"=T19 "Water Valve", "Open/Close (F:Close)"=w460, "error in (no error)"=w456, "Test Type"=w451, "Number Of Cycles"=w450, "Cycle Time (mS)"=w449) -> ("error out"=w455:errorcluster)  [unwired: 4 in, 2 out]
              }
            }
            n213 = call <vilib>:"Add State(s) to Queue__jki_lib_state_machine.vi"("State(s) in (\"\")"=w447) -> ("States Out"=w446:string)  [unwired: 14 in]
          }
          event Value Change {
            n214 = event-data() -> ("NewVal"=w462:bool)  [unwired: 1 in, 2 out]
            n215 = case shown="True" w462 {
              tunnel: w465 -> [_ w478]
              tunnel: w464 -> [w468 w476]
              tunnel: [w468 w475] -> w463
              tunnel: w462 -> [_ w473]
              frame False {
              }
              frame True {
                n216 = local read "Number of ON/OFF Cycles"() -> (w470:i32)
                n217 = local read "Agilent Semaphore"() -> (w479:T1[])
                n218 = local read "Valve ON Time (mS)"() -> (w469:u32)
                n219 = Unbundle By Name(w478) -> ("Agilent Switches"=w477:T2[])
                n220 = local read "Test Type"() -> (w471:T12)
                n221 = Number To Decimal String(number=18) -> (decimal integer string=w481:string)  [unwired: 1 in]
                n222 = Not(x=w473) -> (.not. x?=w480:bool)
                n223 = call "WILT Agilent Valve Control.vi"("Station In"=w481, "Agilent Channels In"=w477, "Semaphore"=w479, "Search"=T19 "Water Valve", "Open/Close (F:Close)"=w480, "error in (no error)"=w476, "Test Type"=w471, "Number Of Cycles"=w470, "Cycle Time (mS)"=w469) -> ("error out"=w475:errorcluster)  [unwired: 4 in, 2 out]
              }
            }
            n224 = call <vilib>:"Add State(s) to Queue__jki_lib_state_machine.vi"("State(s) in (\"\")"=w467) -> ("States Out"=w466:string)  [unwired: 14 in]
          }
          event Value Change {
            n225 = event-data() -> ("NewVal"=w482:bool)  [unwired: 1 in, 2 out]
            n226 = case shown="True" w482 {
              tunnel: w485 -> [_ w498]
              tunnel: w484 -> [w488 w496]
              tunnel: [w488 w495] -> w483
              tunnel: w482 -> [_ w493]
              frame False {
              }
              frame True {
                n227 = local read "Number of ON/OFF Cycles"() -> (w490:i32)
                n228 = local read "Valve ON Time (mS)"() -> (w489:u32)
                n229 = local read "Agilent Semaphore"() -> (w499:T1[])
                n230 = Unbundle By Name(w498) -> ("Agilent Switches"=w497:T2[])
                n231 = local read "Test Type"() -> (w491:T12)
                n232 = Number To Decimal String(number=19) -> (decimal integer string=w501:string)  [unwired: 1 in]
                n233 = Not(x=w493) -> (.not. x?=w500:bool)
                n234 = call "WILT Agilent Valve Control.vi"("Station In"=w501, "Agilent Channels In"=w497, "Semaphore"=w499, "Search"=T19 "Water Valve", "Open/Close (F:Close)"=w500, "error in (no error)"=w496, "Test Type"=w491, "Number Of Cycles"=w490, "Cycle Time (mS)"=w489) -> ("error out"=w495:errorcluster)  [unwired: 4 in, 2 out]
              }
            }
            n235 = call <vilib>:"Add State(s) to Queue__jki_lib_state_machine.vi"("State(s) in (\"\")"=w487) -> ("States Out"=w486:string)  [unwired: 14 in]
          }
          event Value Change {
            n236 = event-data() -> ("NewVal"=w502:bool)  [unwired: 1 in, 2 out]
            n237 = case shown="True" w502 {
              tunnel: w505 -> [_ w518]
              tunnel: w504 -> [w508 w516]
              tunnel: [w508 w515] -> w503
              tunnel: w502 -> [_ w513]
              frame False {
              }
              frame True {
                n238 = local read "Number of ON/OFF Cycles"() -> (w510:i32)
                n239 = local read "Valve ON Time (mS)"() -> (w509:u32)
                n240 = local read "Agilent Semaphore"() -> (w519:T1[])
                n241 = Unbundle By Name(w518) -> ("Agilent Switches"=w517:T2[])
                n242 = local read "Test Type"() -> (w511:T12)
                n243 = Number To Decimal String(number=20) -> (decimal integer string=w521:string)  [unwired: 1 in]
                n244 = Not(x=w513) -> (.not. x?=w520:bool)
                n245 = call "WILT Agilent Valve Control.vi"("Station In"=w521, "Agilent Channels In"=w517, "Semaphore"=w519, "Search"=T19 "Water Valve", "Open/Close (F:Close)"=w520, "error in (no error)"=w516, "Test Type"=w511, "Number Of Cycles"=w510, "Cycle Time (mS)"=w509) -> ("error out"=w515:errorcluster)  [unwired: 4 in, 2 out]
              }
            }
            n246 = call <vilib>:"Add State(s) to Queue__jki_lib_state_machine.vi"("State(s) in (\"\")"=w507) -> ("States Out"=w506:string)  [unwired: 14 in]
          }
          event Value Change {
            n247 = event-data() -> ("NewVal"=w522:bool)  [unwired: 1 in, 2 out]
            n248 = case shown="True" w522 {
              tunnel: w525 -> [_ w538]
              tunnel: w524 -> [w528 w536]
              tunnel: [w528 w535] -> w523
              tunnel: w522 -> [_ w533]
              frame False {
              }
              frame True {
                n249 = local read "Number of ON/OFF Cycles"() -> (w530:i32)
                n250 = local read "Valve ON Time (mS)"() -> (w529:u32)
                n251 = local read "Agilent Semaphore"() -> (w539:T1[])
                n252 = Unbundle By Name(w538) -> ("Agilent Switches"=w537:T2[])
                n253 = local read "Test Type"() -> (w531:T12)
                n254 = Number To Decimal String(number=21) -> (decimal integer string=w541:string)  [unwired: 1 in]
                n255 = Not(x=w533) -> (.not. x?=w540:bool)
                n256 = call "WILT Agilent Valve Control.vi"("Station In"=w541, "Agilent Channels In"=w537, "Semaphore"=w539, "Search"=T19 "Water Valve", "Open/Close (F:Close)"=w540, "error in (no error)"=w536, "Test Type"=w531, "Number Of Cycles"=w530, "Cycle Time (mS)"=w529) -> ("error out"=w535:errorcluster)  [unwired: 4 in, 2 out]
              }
            }
            n257 = call <vilib>:"Add State(s) to Queue__jki_lib_state_machine.vi"("State(s) in (\"\")"=w527) -> ("States Out"=w526:string)  [unwired: 14 in]
          }
          event Value Change {
            n258 = event-data() -> ("NewVal"=w542:bool)  [unwired: 1 in, 2 out]
            n259 = case shown="True" w542 {
              tunnel: w545 -> [_ w558]
              tunnel: w544 -> [w548 w556]
              tunnel: [w548 w555] -> w543
              tunnel: w542 -> [_ w553]
              frame False {
              }
              frame True {
                n260 = local read "Number of ON/OFF Cycles"() -> (w550:i32)
                n261 = local read "Valve ON Time (mS)"() -> (w549:u32)
                n262 = local read "Agilent Semaphore"() -> (w559:T1[])
                n263 = Unbundle By Name(w558) -> ("Agilent Switches"=w557:T2[])
                n264 = local read "Test Type"() -> (w551:T12)
                n265 = Number To Decimal String(number=22) -> (decimal integer string=w561:string)  [unwired: 1 in]
                n266 = Not(x=w553) -> (.not. x?=w560:bool)
                n267 = call "WILT Agilent Valve Control.vi"("Station In"=w561, "Agilent Channels In"=w557, "Semaphore"=w559, "Search"=T19 "Water Valve", "Open/Close (F:Close)"=w560, "error in (no error)"=w556, "Test Type"=w551, "Number Of Cycles"=w550, "Cycle Time (mS)"=w549) -> ("error out"=w555:errorcluster)  [unwired: 4 in, 2 out]
              }
            }
            n268 = call <vilib>:"Add State(s) to Queue__jki_lib_state_machine.vi"("State(s) in (\"\")"=w547) -> ("States Out"=w546:string)  [unwired: 14 in]
          }
          event Value Change {
            n269 = event-data() -> ("NewVal"=w562:bool)  [unwired: 1 in, 2 out]
            n270 = case shown="True" w562 {
              tunnel: w565 -> [_ w578]
              tunnel: w564 -> [w568 w576]
              tunnel: [w568 w575] -> w563
              tunnel: w562 -> [_ w573]
              frame False {
              }
              frame True {
                n271 = local read "Number of ON/OFF Cycles"() -> (w570:i32)
                n272 = local read "Valve ON Time (mS)"() -> (w569:u32)
                n273 = local read "Agilent Semaphore"() -> (w579:T1[])
                n274 = Unbundle By Name(w578) -> ("Agilent Switches"=w577:T2[])
                n275 = local read "Test Type"() -> (w571:T12)
                n276 = Number To Decimal String(number=23) -> (decimal integer string=w581:string)  [unwired: 1 in]
                n277 = Not(x=w573) -> (.not. x?=w580:bool)
                n278 = call "WILT Agilent Valve Control.vi"("Station In"=w581, "Agilent Channels In"=w577, "Semaphore"=w579, "Search"=T19 "Water Valve", "Open/Close (F:Close)"=w580, "error in (no error)"=w576, "Test Type"=w571, "Number Of Cycles"=w570, "Cycle Time (mS)"=w569) -> ("error out"=w575:errorcluster)  [unwired: 4 in, 2 out]
              }
            }
            n279 = call <vilib>:"Add State(s) to Queue__jki_lib_state_machine.vi"("State(s) in (\"\")"=w567) -> ("States Out"=w566:string)  [unwired: 14 in]
          }
          event Value Change {
            n280 = event-data() -> ("NewVal"=w582:bool)  [unwired: 1 in, 2 out]
            n281 = case shown="True" w582 {
              tunnel: w585 -> [_ w598]
              tunnel: w584 -> [w588 w596]
              tunnel: [w588 w595] -> w583
              tunnel: w582 -> [_ w593]
              frame False {
              }
              frame True {
                n282 = local read "Number of ON/OFF Cycles"() -> (w590:i32)
                n283 = local read "Valve ON Time (mS)"() -> (w589:u32)
                n284 = local read "Agilent Semaphore"() -> (w599:T1[])
                n285 = Unbundle By Name(w598) -> ("Agilent Switches"=w597:T2[])
                n286 = local read "Test Type"() -> (w591:T12)
                n287 = Number To Decimal String(number=24) -> (decimal integer string=w601:string)  [unwired: 1 in]
                n288 = Not(x=w593) -> (.not. x?=w600:bool)
                n289 = call "WILT Agilent Valve Control.vi"("Station In"=w601, "Agilent Channels In"=w597, "Semaphore"=w599, "Search"=T19 "Water Valve", "Open/Close (F:Close)"=w600, "error in (no error)"=w596, "Test Type"=w591, "Number Of Cycles"=w590, "Cycle Time (mS)"=w589) -> ("error out"=w595:errorcluster)  [unwired: 4 in, 2 out]
              }
            }
            n290 = call <vilib>:"Add State(s) to Queue__jki_lib_state_machine.vi"("State(s) in (\"\")"=w587) -> ("States Out"=w586:string)  [unwired: 14 in]
          }
          event Value Change {
            n291 = event-data() -> ("NewVal"=w602:bool)  [unwired: 1 in, 2 out]
            n292 = case shown="True" w602 {
              tunnel: w605 -> [_ w618]
              tunnel: w604 -> [w608 w616]
              tunnel: [w608 w615] -> w603
              tunnel: w602 -> [_ w613]
              frame False {
              }
              frame True {
                n293 = local read "Number of ON/OFF Cycles"() -> (w610:i32)
                n294 = local read "Valve ON Time (mS)"() -> (w609:u32)
                n295 = local read "Agilent Semaphore"() -> (w619:T1[])
                n296 = Unbundle By Name(w618) -> ("Agilent Switches"=w617:T2[])
                n297 = local read "Test Type"() -> (w611:T12)
                n298 = Number To Decimal String(number=25) -> (decimal integer string=w621:string)  [unwired: 1 in]
                n299 = Not(x=w613) -> (.not. x?=w620:bool)
                n300 = call "WILT Agilent Valve Control.vi"("Station In"=w621, "Agilent Channels In"=w617, "Semaphore"=w619, "Search"=T19 "Water Valve", "Open/Close (F:Close)"=w620, "error in (no error)"=w616, "Test Type"=w611, "Number Of Cycles"=w610, "Cycle Time (mS)"=w609) -> ("error out"=w615:errorcluster)  [unwired: 4 in, 2 out]
              }
            }
            n301 = call <vilib>:"Add State(s) to Queue__jki_lib_state_machine.vi"("State(s) in (\"\")"=w607) -> ("States Out"=w606:string)  [unwired: 14 in]
          }
          event Value Change {
            n302 = event-data() -> ("NewVal"=w622:bool)  [unwired: 1 in, 2 out]
            n303 = case shown="True" w622 {
              tunnel: w625 -> [_ w638]
              tunnel: [w628 w636] -> w624
              tunnel: w622 -> [_ w634]
              tunnel: w623 -> [w628 w632]
              frame False {
              }
              frame True {
                n304 = local read "Number of ON/OFF Cycles"() -> (w630:i32)
                n305 = local read "Valve ON Time (mS)"() -> (w629:u32)
                n306 = local read "Agilent Semaphore"() -> (w639:T1[])
                n307 = Unbundle By Name(w638) -> ("Agilent Switches"=w637:T2[])
                n308 = local read "Test Type"() -> (w631:T12)
                n309 = Number To Decimal String(number=26) -> (decimal integer string=w641:string)  [unwired: 1 in]
                n310 = Not(x=w634) -> (.not. x?=w640:bool)
                n311 = call "WILT Agilent Valve Control.vi"("Station In"=w641, "Agilent Channels In"=w637, "Semaphore"=w639, "Search"=T19 "Water Valve", "Open/Close (F:Close)"=w640, "error in (no error)"=w632, "Test Type"=w631, "Number Of Cycles"=w630, "Cycle Time (mS)"=w629) -> ("error out"=w636:errorcluster)  [unwired: 4 in, 2 out]
              }
            }
            n312 = call <vilib>:"Add State(s) to Queue__jki_lib_state_machine.vi"("State(s) in (\"\")"=w627) -> ("States Out"=w626:string)  [unwired: 14 in]
          }
          event Value Change {
            n313 = event-data() -> ("NewVal"=w642:bool)  [unwired: 1 in, 2 out]
            n314 = case shown="True" w642 {
              tunnel: w645 -> [_ w658]
              tunnel: w644 -> [w648 w656]
              tunnel: [w648 w655] -> w643
              tunnel: w642 -> [_ w653]
              frame False {
              }
              frame True {
                n315 = local read "Number of ON/OFF Cycles"() -> (w650:i32)
                n316 = local read "Agilent Semaphore"() -> (w659:T1[])
                n317 = local read "Valve ON Time (mS)"() -> (w649:u32)
                n318 = Unbundle By Name(w658) -> ("Agilent Switches"=w657:T2[])
                n319 = local read "Test Type"() -> (w651:T12)
                n320 = Number To Decimal String(number=27) -> (decimal integer string=w661:string)  [unwired: 1 in]
                n321 = Not(x=w653) -> (.not. x?=w660:bool)
                n322 = call "WILT Agilent Valve Control.vi"("Station In"=w661, "Agilent Channels In"=w657, "Semaphore"=w659, "Search"=T19 "Water Valve", "Open/Close (F:Close)"=w660, "error in (no error)"=w656, "Test Type"=w651, "Number Of Cycles"=w650, "Cycle Time (mS)"=w649) -> ("error out"=w655:errorcluster)  [unwired: 4 in, 2 out]
              }
            }
            n323 = call <vilib>:"Add State(s) to Queue__jki_lib_state_machine.vi"("State(s) in (\"\")"=w647) -> ("States Out"=w646:string)  [unwired: 14 in]
          }
          event Value Change {
            n324 = event-data() -> ("NewVal"=w662:bool)  [unwired: 1 in, 2 out]
            n325 = case shown="True" w662 {
              tunnel: w665 -> [_ w678]
              tunnel: w664 -> [w668 w676]
              tunnel: [w668 w675] -> w663
              tunnel: w662 -> [_ w673]
              frame False {
              }
              frame True {
                n326 = local read "Number of ON/OFF Cycles"() -> (w670:i32)
                n327 = local read "Valve ON Time (mS)"() -> (w669:u32)
                n328 = local read "Agilent Semaphore"() -> (w679:T1[])
                n329 = Unbundle By Name(w678) -> ("Agilent Switches"=w677:T2[])
                n330 = local read "Test Type"() -> (w671:T12)
                n331 = Number To Decimal String(number=28) -> (decimal integer string=w681:string)  [unwired: 1 in]
                n332 = Not(x=w673) -> (.not. x?=w680:bool)
                n333 = call "WILT Agilent Valve Control.vi"("Station In"=w681, "Agilent Channels In"=w677, "Semaphore"=w679, "Search"=T19 "Water Valve", "Open/Close (F:Close)"=w680, "error in (no error)"=w676, "Test Type"=w671, "Number Of Cycles"=w670, "Cycle Time (mS)"=w669) -> ("error out"=w675:errorcluster)  [unwired: 4 in, 2 out]
              }
            }
            n334 = call <vilib>:"Add State(s) to Queue__jki_lib_state_machine.vi"("State(s) in (\"\")"=w667) -> ("States Out"=w666:string)  [unwired: 14 in]
          }
          event Value Change {
            n335 = event-data() -> ("NewVal"=w682:bool)  [unwired: 1 in, 2 out]
            n336 = case shown="True" w682 {
              tunnel: w685 -> [_ w698]
              tunnel: w684 -> [w688 w696]
              tunnel: [w688 w695] -> w683
              tunnel: w682 -> [_ w693]
              frame False {
              }
              frame True {
                n337 = local read "Number of ON/OFF Cycles"() -> (w690:i32)
                n338 = local read "Valve ON Time (mS)"() -> (w689:u32)
                n339 = local read "Agilent Semaphore"() -> (w699:T1[])
                n340 = Unbundle By Name(w698) -> ("Agilent Switches"=w697:T2[])
                n341 = local read "Test Type"() -> (w691:T12)
                n342 = Number To Decimal String(number=29) -> (decimal integer string=w701:string)  [unwired: 1 in]
                n343 = Not(x=w693) -> (.not. x?=w700:bool)
                n344 = call "WILT Agilent Valve Control.vi"("Station In"=w701, "Agilent Channels In"=w697, "Semaphore"=w699, "Search"=T19 "Water Valve", "Open/Close (F:Close)"=w700, "error in (no error)"=w696, "Test Type"=w691, "Number Of Cycles"=w690, "Cycle Time (mS)"=w689) -> ("error out"=w695:errorcluster)  [unwired: 4 in, 2 out]
              }
            }
            n345 = call <vilib>:"Add State(s) to Queue__jki_lib_state_machine.vi"("State(s) in (\"\")"=w687) -> ("States Out"=w686:string)  [unwired: 14 in]
          }
          event Value Change {
            n346 = event-data() -> ("NewVal"=w702:bool)  [unwired: 1 in, 2 out]
            n347 = case shown="False" w702 {
              tunnel: w705 -> [_ w718]
              tunnel: w704 -> [w708 w716]
              tunnel: [w708 w715] -> w703
              tunnel: w702 -> [_ w713]
              frame False {
              }
              frame True {
                n348 = local read "Number of ON/OFF Cycles"() -> (w710:i32)
                n349 = local read "Valve ON Time (mS)"() -> (w709:u32)
                n350 = local read "Agilent Semaphore"() -> (w719:T1[])
                n351 = Unbundle By Name(w718) -> ("Agilent Switches"=w717:T2[])
                n352 = local read "Test Type"() -> (w711:T12)
                n353 = Number To Decimal String(number=30) -> (decimal integer string=w721:string)  [unwired: 1 in]
                n354 = Not(x=w713) -> (.not. x?=w720:bool)
                n355 = call "WILT Agilent Valve Control.vi"("Station In"=w721, "Agilent Channels In"=w717, "Semaphore"=w719, "Search"=T19 "Water Valve", "Open/Close (F:Close)"=w720, "error in (no error)"=w716, "Test Type"=w711, "Number Of Cycles"=w710, "Cycle Time (mS)"=w709) -> ("error out"=w715:errorcluster)  [unwired: 4 in, 2 out]
              }
            }
            n356 = call <vilib>:"Add State(s) to Queue__jki_lib_state_machine.vi"("State(s) in (\"\")"=w707) -> ("States Out"=w706:string)  [unwired: 14 in]
          }
          event Value Change {
            n357 = event-data() -> ("NewVal"=w722:bool)  [unwired: 1 in, 2 out]
            n358 = case shown="False" w722 {
              tunnel: w725 -> [_ w738]
              tunnel: w724 -> [w728 w736]
              tunnel: [w728 w735] -> w723
              tunnel: w722 -> [_ w733]
              frame False {
              }
              frame True {
                n359 = local read "Number of ON/OFF Cycles"() -> (w730:i32)
                n360 = local read "Agilent Semaphore"() -> (w739:T1[])
                n361 = local read "Valve ON Time (mS)"() -> (w729:u32)
                n362 = Unbundle By Name(w738) -> ("Agilent Switches"=w737:T2[])
                n363 = local read "Test Type"() -> (w731:T12)
                n364 = Number To Decimal String(number=31) -> (decimal integer string=w741:string)  [unwired: 1 in]
                n365 = Not(x=w733) -> (.not. x?=w740:bool)
                n366 = call "WILT Agilent Valve Control.vi"("Station In"=w741, "Agilent Channels In"=w737, "Semaphore"=w739, "Search"=T19 "Water Valve", "Open/Close (F:Close)"=w740, "error in (no error)"=w736, "Test Type"=w731, "Number Of Cycles"=w730, "Cycle Time (mS)"=w729) -> ("error out"=w735:errorcluster)  [unwired: 4 in, 2 out]
              }
            }
            n367 = call <vilib>:"Add State(s) to Queue__jki_lib_state_machine.vi"("State(s) in (\"\")"=w727) -> ("States Out"=w726:string)  [unwired: 14 in]
          }
          event Value Change {
